vi "Convert_ERDs_Version_ARG.vi"(0 "New Header?":bool, 2 "ERD Name":string[](array[string]), 5 "All_Bundled_Data_Brass":T1, 7 "Array":T8[](array[typedef]) {"ERD Number" format="%.0x"}, 11 "Error In":errorcluster) -> (6 "All_Bundled_Data_Brass 2":T1, 15 "Error Out":errorcluster)   [LabVIEW 2021]
doc: "This VI parses the data from ERDs in correct format, units, etc. It handles all hex to dec conversions, hex to enum, and hex to boolean conversions.\n\nIf Raw Data from ERD is blank string, then it will output values from shift register."
uses:
  Common/LabVIEW GEA2 Toolkit/GEA3/type defs/ERD Read Data Out.ctl
  Type defs/All_Bundled_Data_ARG.ctl
  Common/type defs/Version.ctl
  Common/type defs/CSV_File_String_Arrays.ctl
  Common/type defs/Fault Table Array.ctl
  Common/type defs/Fault_Table_Info.ctl
  Common/type defs/BootloaderVersion.ctl
  Type defs/ERD_Always_Show_ARG.ctl
panel:
  out "Numeric":i32
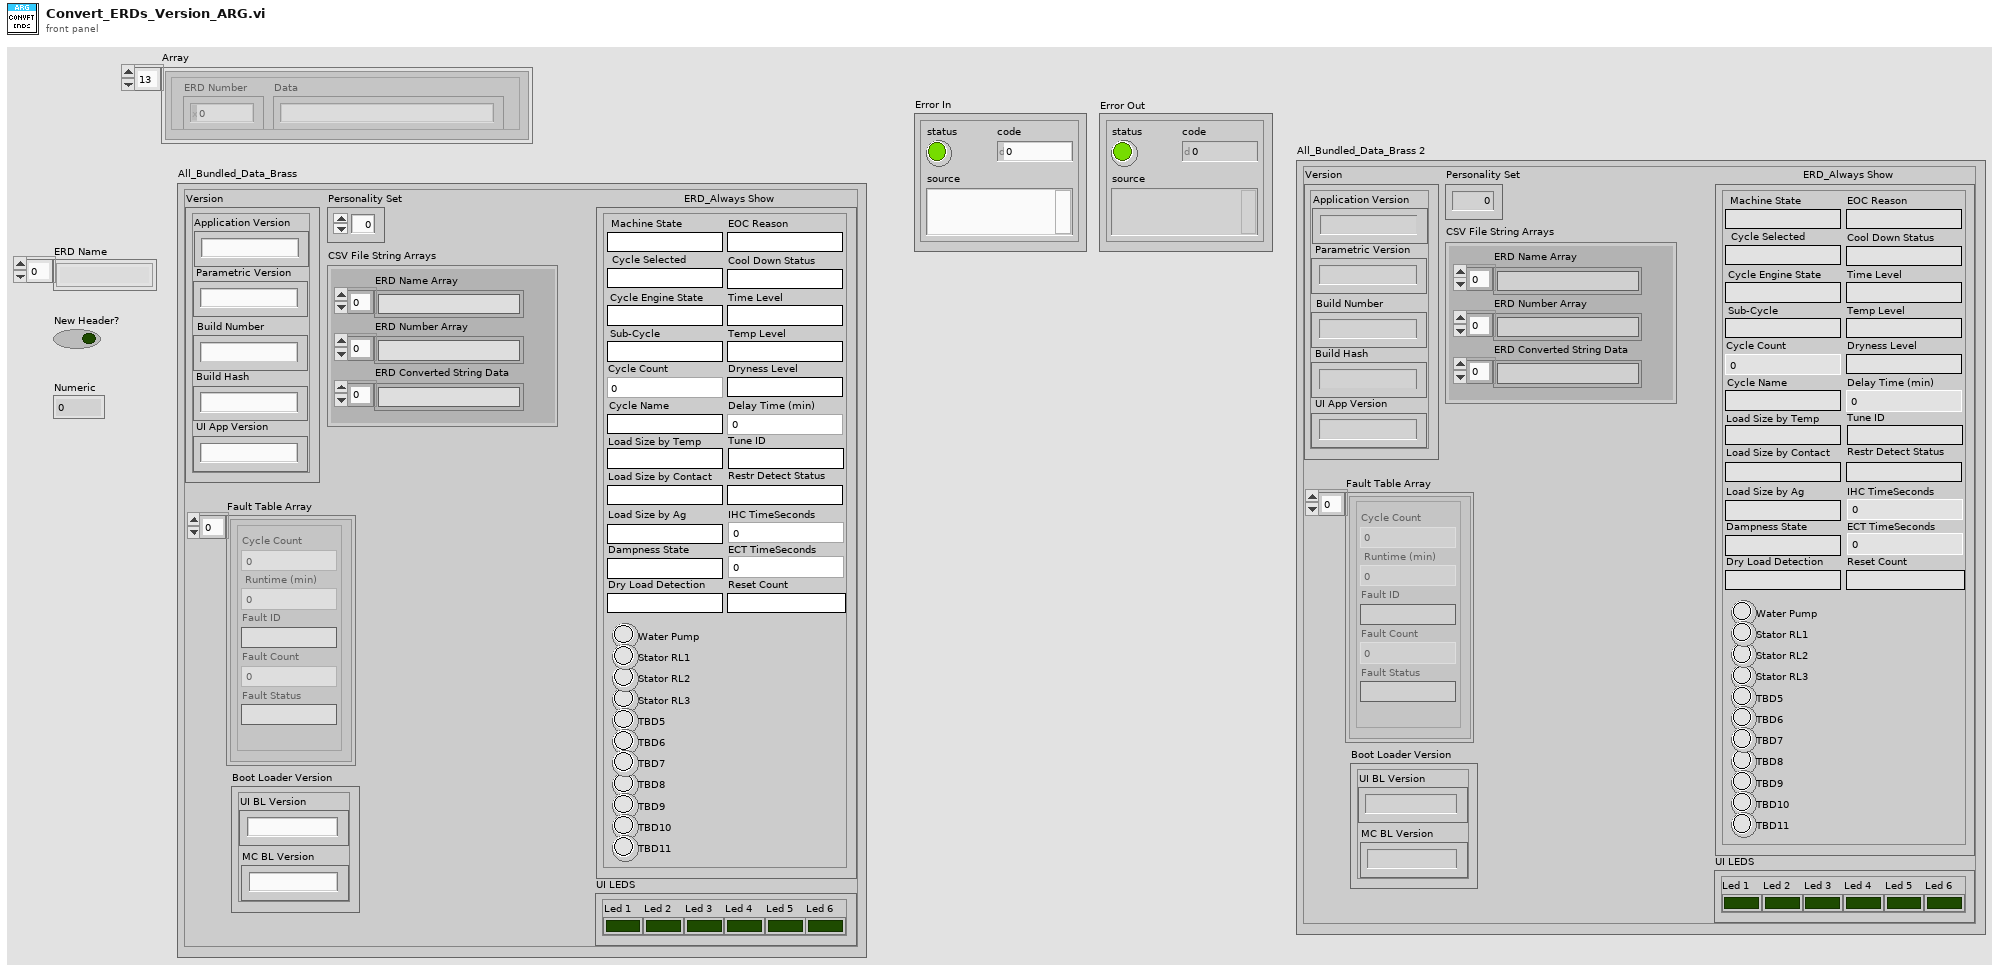
[diagram p1: front panel]
types:
  T1 = typedef "All_Bundled_Data_ARG.ctl" = cluster{"Version":T2, "Personality Set":u8, "CSV File String Arrays":T3, "Fault Table Array ":T4, "Boot Loader Version":T6, "ERD_Always Show":T7, "UI LEDS":cluster{"Led 1":bool, "Led 2":bool, "Led 3":bool, "Led 4":bool, "Led 5":bool, "Led 6":bool}}
  T2 = typedef "Version.ctl" = cluster{"Build Number":string, "Build Hash ":string, "Application Version":string, "Parametric Version":string, "UI App Version":string}
  T3 = typedef "CSV_File_String_Arrays.ctl" = cluster{"ERD Number Array":string[], "ERD Name Array":string[], "ERD Converted String Data":string[]}
  T4 = typedef "Fault Table Array.ctl" = T5[]
  T5 = typedef "Fault_Table_Info.ctl" = cluster{"Cycle Count":u32, " Runtime (min) ":u32, "Fault Status":string, "Fault ID":string, "Fault Count":u16}
  T6 = typedef "BootloaderVersion.ctl" = cluster{"UI BL Version":string, "MC BL Version":string}
  T7 = typedef "ERD_Always_Show_ARG.ctl" = cluster{"Machine State":string, "Cycle Selected":string, "Cycle Engine State":string, "Cycle Count":u32, "Temp Level":string, "Dryness Level":string, "Time Level":string, "Delay Time (min)":u16, "Sub-Cycle":string, "Cycle Name":string, "Tune ID":string, "Restr Detect Status":string, "Load Size by Contact":string, "Load Size by Temp":string, "EOC Reason":string, "Reset Count":string, "Dampness State":string, "Stator RL3":bool, "TBD5":bool, "TBD6":bool, "Water Pump":bool, "Stator RL2":bool, "Cool Down Status":string, "TBD8":bool, "TBD9":bool, "TBD10":bool, "TBD11":bool, "TBD7":bool, "Stator RL1":bool, "IHC TimeSeconds":u32, "ECT TimeSeconds ":u32, "Load Size by Ag":string, "Dry Load Detection":string}
  T8 = typedef "ERD Read Data Out.ctl" = cluster{"ERD Number":u16, "Data":string}
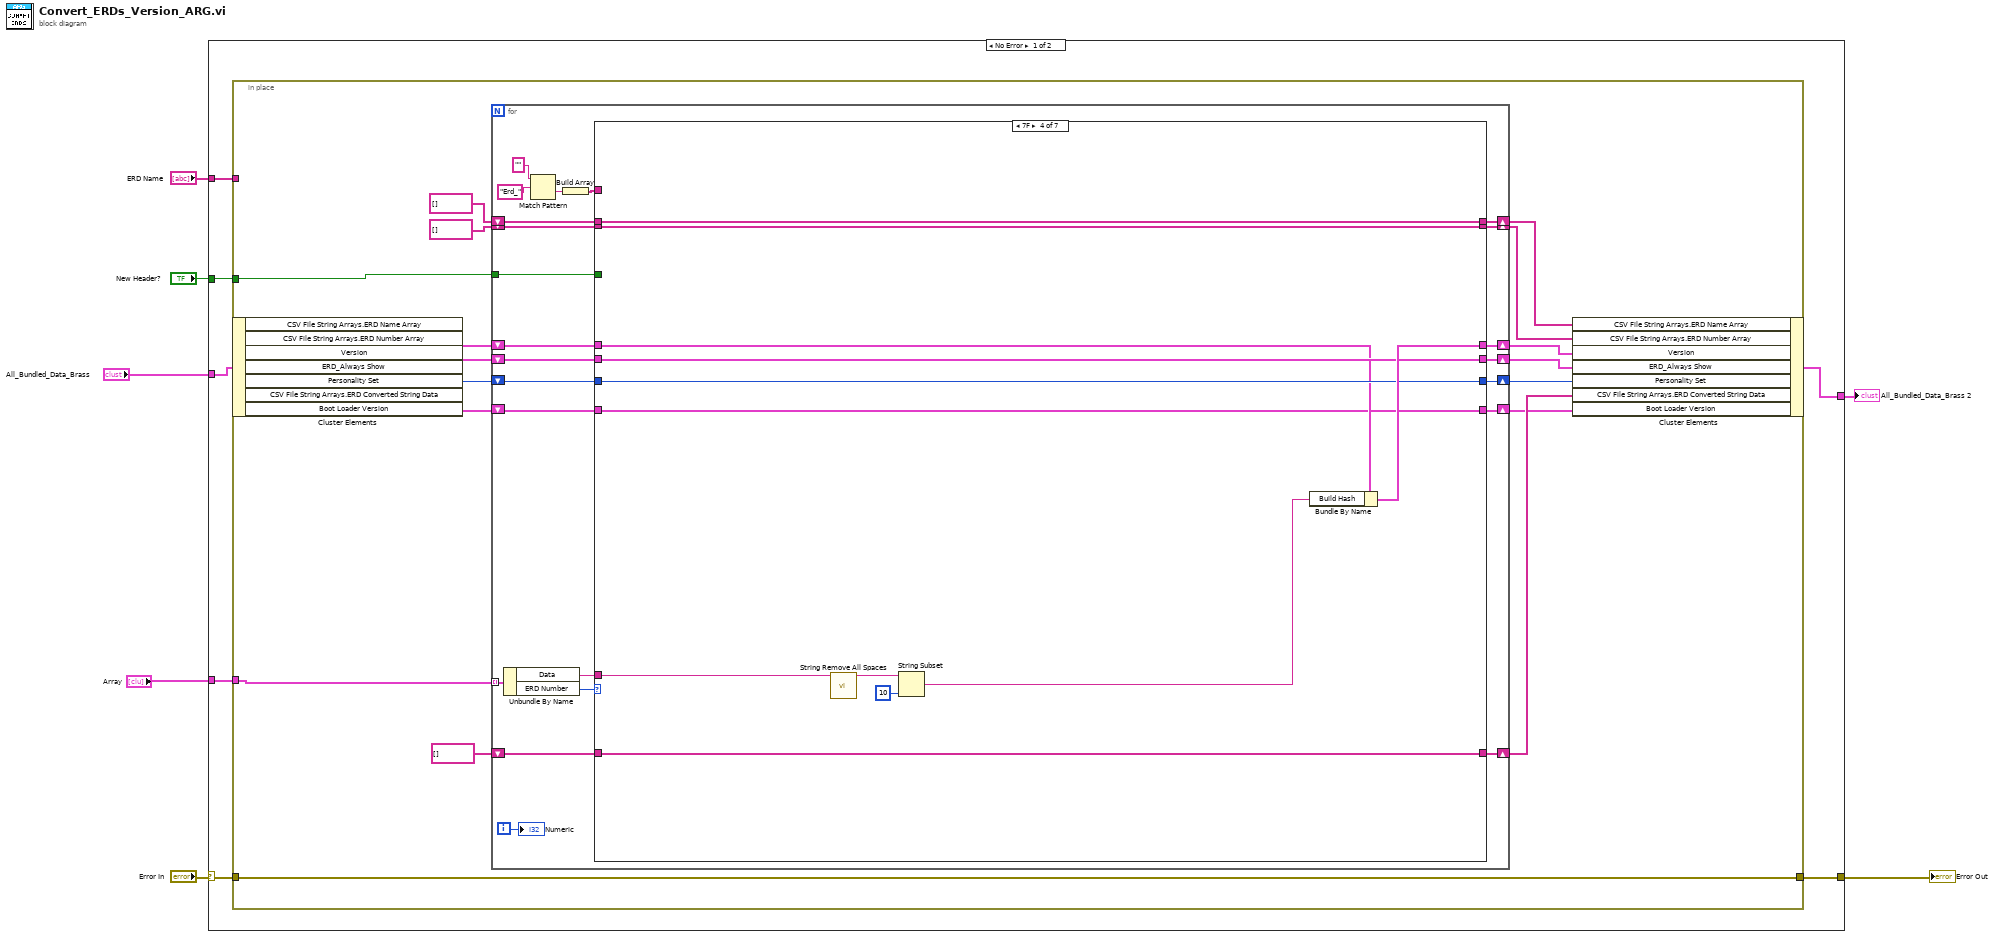
[diagram p0: block diagram]
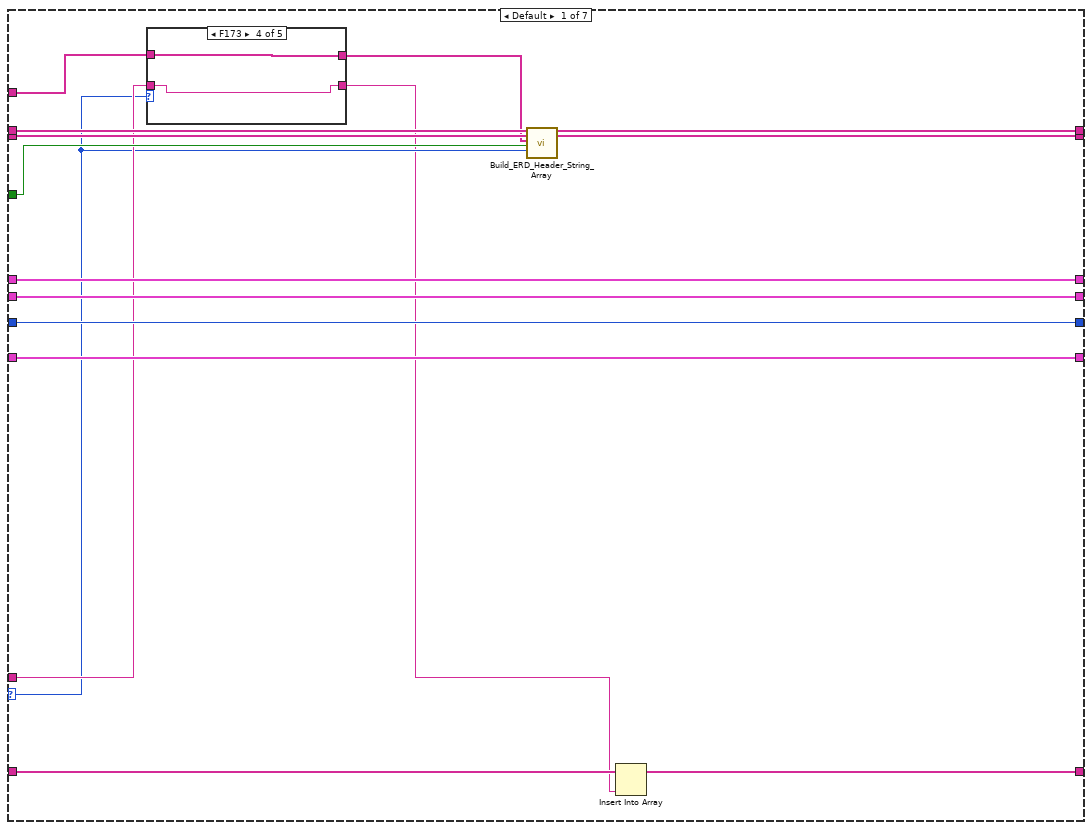
[diagram p2: hidden frame]
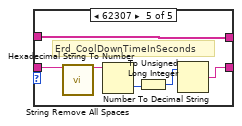
[diagram p6: hidden frame]
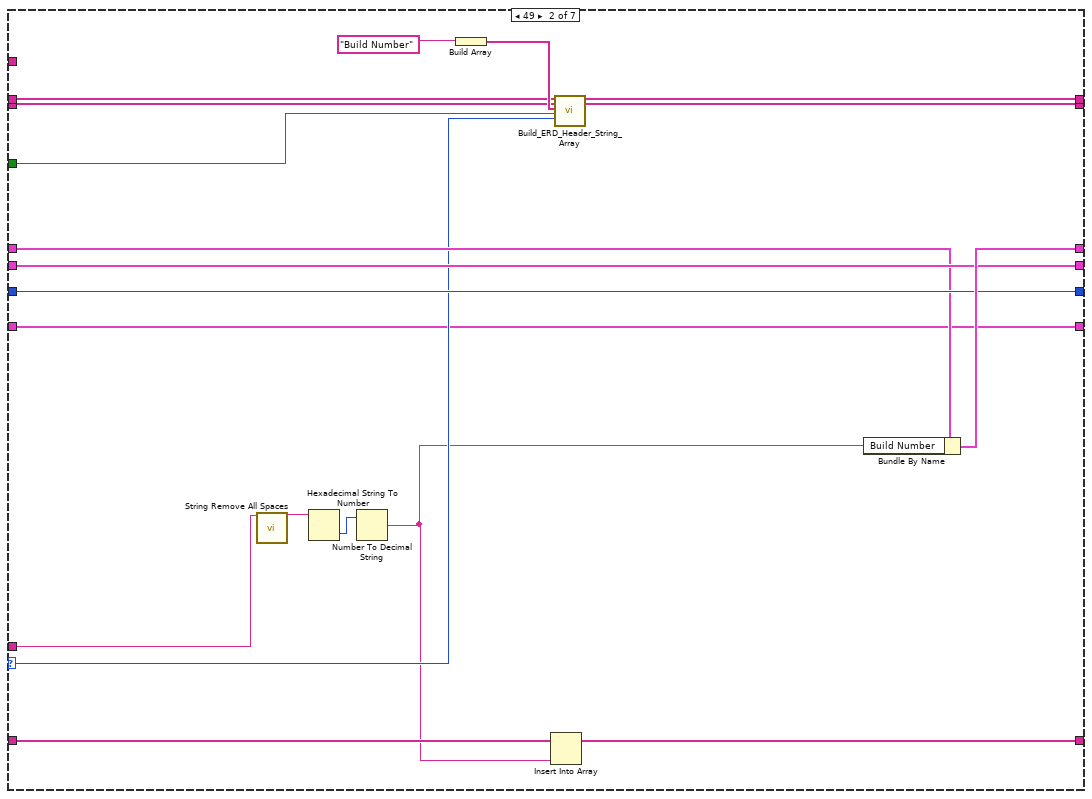
[diagram p7: hidden frame]
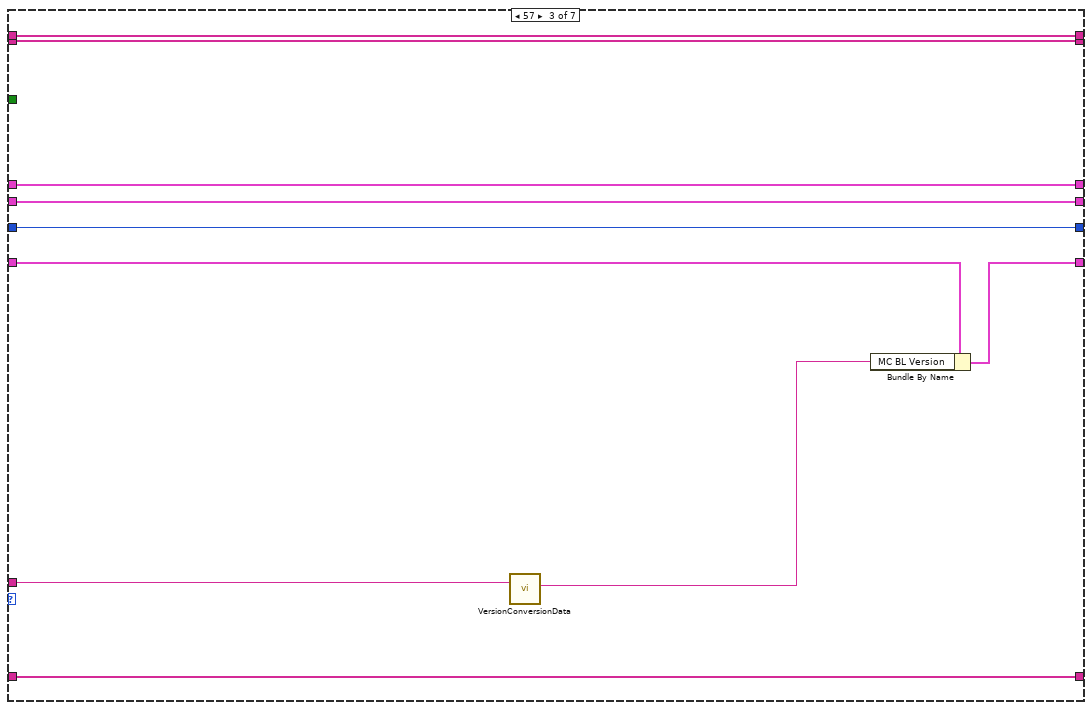
[diagram p8: hidden frame]
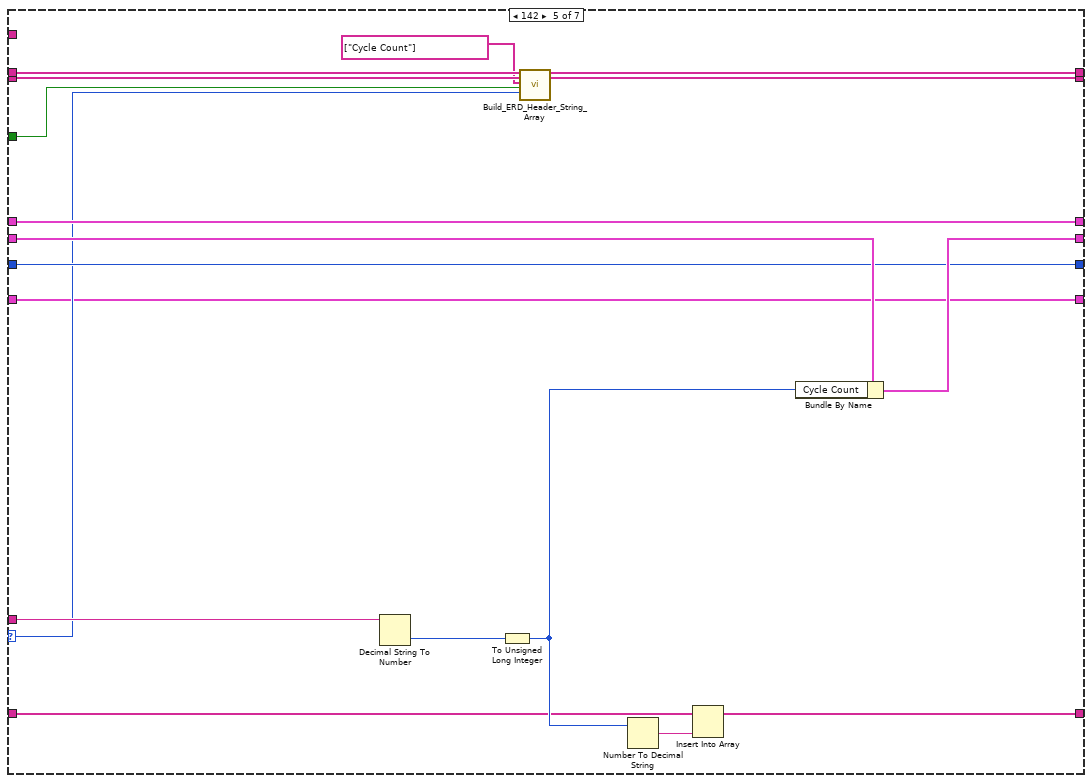
[diagram p9: hidden frame]
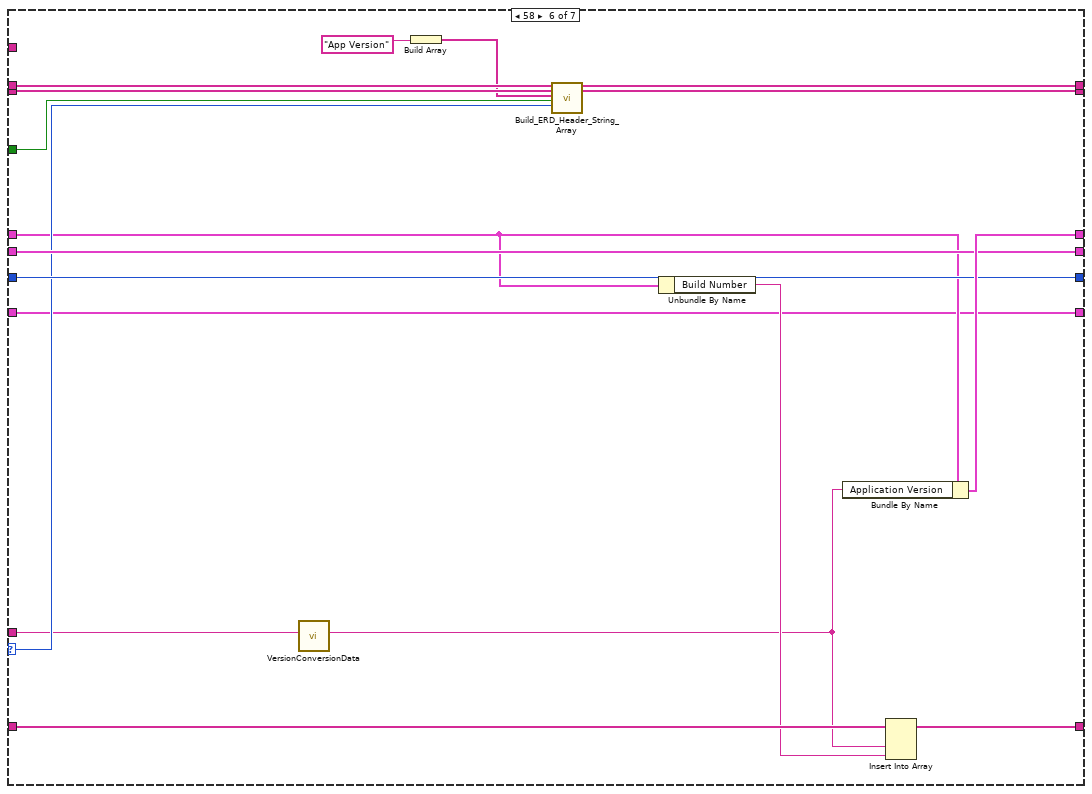
[diagram p10: hidden frame]
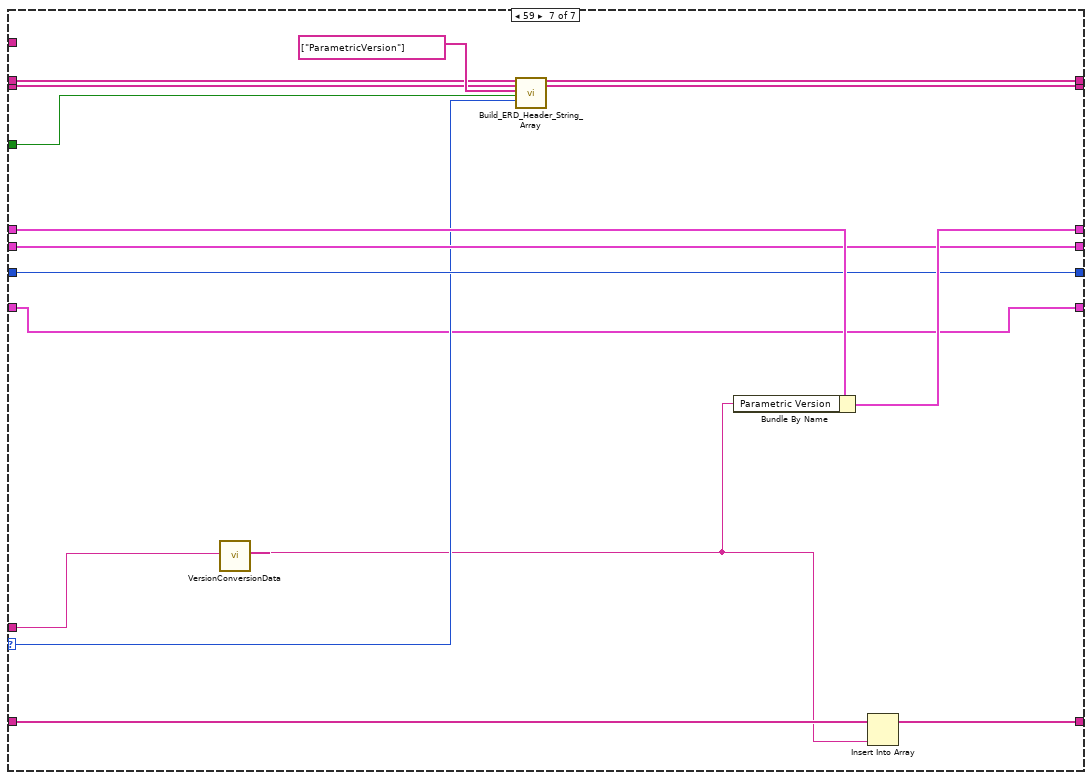
[diagram p11: hidden frame]
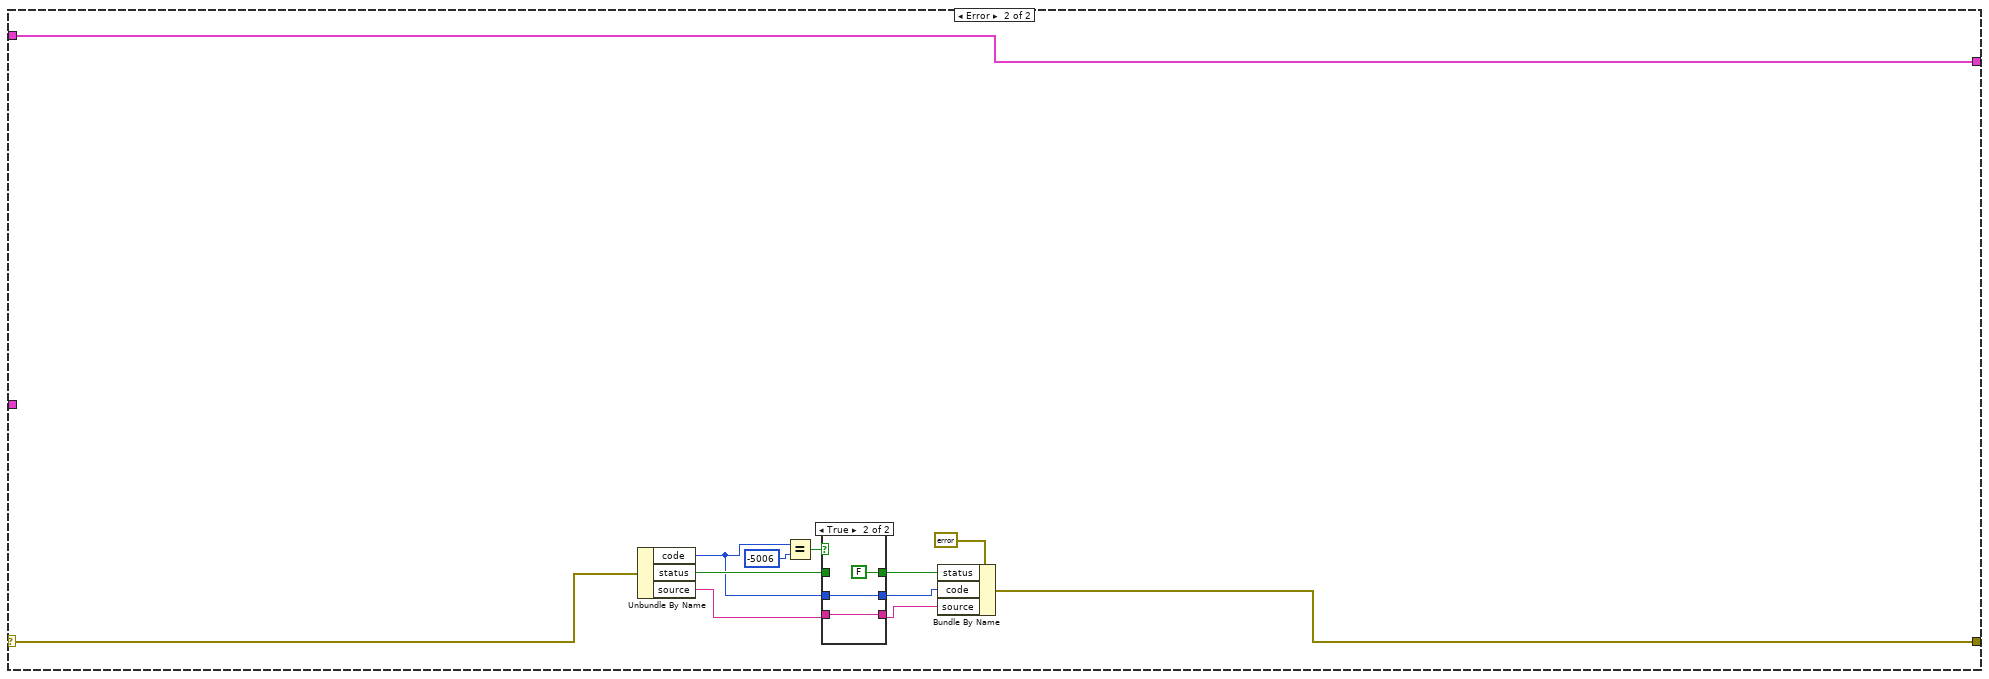
[diagram p12: hidden frame]
diagram:
  n1 = case shown="No Error" "Error In" {
    selector: "Error In" -> [w11 w180]
    tunnel: "Array" -> [w14 _]
    tunnel: [w12 w179] -> w5
    tunnel: "All_Bundled_Data_Brass" -> [w13 w178]
    tunnel: [w10 w178] -> w1
    tunnel: "New Header?" -> [w9 _]
    tunnel: "ERD Name" -> [w8 _]
    frame No Error {
      n2 = in-place {
        in-place-border: w14 -> [w16]
        in-place-border: [w15] -> w12
        in-place-border: w11 -> [w15]
        in-place-border: w9 -> [w24]
        in-place-border: w8 -> [_]
        n3 = in-place-cluster #1(w13) -> ("Version"=w30:T2, "ERD_Always Show"=w31:T7, "Personality Set"=w27:u8, "Boot Loader Version"=w18:T6)  [unwired: 3 out]
        n4 = for {
          shift-right: [w53] -> w28
          shift-left: w31 -> [w52]
          shift-right: [w50] -> w29
          shift-left: w30 -> [w51]
          shift-right: [w47] -> w26
          shift-left: w27 -> [w48]
          shift-right: [w45] -> w19
          shift-left: string[] [] ("ERD String Data") -> [w46]
          tunnel: w24 -> [w44]
          shift-right: [w40] -> w20
          shift-left: string[] [] ("ERD String Data") -> [w43]
          shift-right: [w41] -> w21
          shift-left: string[] [] ("ERD String Data") -> [w42]
          shift-right: [w37] -> w17
          shift-left: w18 -> [w38]
          tunnel: w16 -> [w33] mode=indexing
          i -> [w39]
          n5 = Unbundle By Name(w33) -> ("Data"=w54:string, "ERD Number"=w49:u16)
          n6 = Match Pattern(string="", regular expression="Erd_") -> (after substring=w34:string)  [unwired: 1 in, 3 out]
          n7 = Build Array(w34) -> (w35:string[])
          n8 = case shown="7F" w49 {
            selector: w49 -> [w56 w94 _ _ w132 w153 w165]
            tunnel: w54 -> [w57 w88 w105 w119 w143 w145 w163]
            tunnel: [w70 w102 w113 w124 w141 w160 w175] -> w53
            tunnel: w52 -> [w70 w102 w113 w124 w142 w160 w175]
            tunnel: w51 -> [w69 w100 w106 w120 w140 w152 w177]
            tunnel: [w69 w103 w106 w125 w140 w161 w176] -> w50
            tunnel: w48 -> [w68 w101 w112 w123 w139 w159 w174]
            tunnel: [w68 w101 w112 w123 w139 w159 w174] -> w47
            tunnel: w46 -> [w66 w98 w109 w115 w137 w148 w169]
            tunnel: [w62 w97 w109 w115 w135 w155 w167] -> w45
            tunnel: w44 -> [w64 w92 _ _ w133 w154 w166]
            tunnel: w43 -> [w65 w96 w110 w121 w138 w149 w170]
            tunnel: w42 -> [w60 w90 w111 w122 w128 w158 w173]
            tunnel: [w61 w89 w111 w122 w127 w157 w172] -> w41
            tunnel: [w63 w95 w110 w121 w136 w156 w168] -> w40
            tunnel: w38 -> [w67 w91 w108 w114 w126 w150 w164]
            tunnel: [w67 w91 w107 w114 w126 w150 w164] -> w37
            tunnel: w35 -> [w58 _ _ _ _ _ _]
            frame Default {
              n9 = case shown="F173" w56 {
                tunnel: [w71 w74 w76 w78 w84] -> w59
                tunnel: w58 -> [w71 w74 w76 w78 w84]
                tunnel: w57 -> [w72 w73 w75 w77 w81]
                tunnel: [w72 w73 w75 w77 w79] -> w55
                frame 0, Default {
                  # "ERDs No Data Conversion"
                }
                frame 65423 {
                  # "Consumer Error Mode"
                }
                frame 55 {
                  # "ServiceModeState"
                }
                frame 61811 {
                }
                frame 62307 {
                  # "Erd_CoolDownTimeInSeconds"
                  n10 = call "String Remove All Spaces.vi"("Input String"=w81) -> ("Spaces Removed"=w82:string)  [unwired: 13 in, 1 out]
                  n11 = Hexadecimal String To Number(string=w82) -> (number=w83:u32)  [unwired: 2 in, 1 out]
                  n12 = To Unsigned Long Integer(number=w83) -> (unsigned 32bit integer=w80:u32)
                  n13 = Number To Decimal String(number=w80) -> (decimal integer string=w79:string)  [unwired: 1 in]
                }
              }
              n14 = call "Build_ERD_Header_String_Array.vi"("ERD Name Array In"=w65, "ERD Number Array In"=w66, "ERD Name List"=w59, "New Header?"=w64, "ERD Number"=w56) -> ("ERD Name Array Out"=w63:string[], "ERD Number Array Out"=w62:string[])  [unwired: 13 in]
              n15 = Insert Into Array(array=w60, new element=w55) -> (w61:string[])  [unwired: 1 in]
            }
            frame 49 {
              n16 = call "String Remove All Spaces.vi"("Input String"=w88) -> ("Spaces Removed"=w87:string)  [unwired: 13 in, 1 out]
              n17 = Hexadecimal String To Number(string=w87) -> (number=w85:u32)  [unwired: 2 in, 1 out]
              n18 = Number To Decimal String(number=w85) -> (decimal integer string=w86:string)  [unwired: 1 in]
              n19 = Build Array("Build Number") -> (w99:string[])
              n20 = Insert Into Array(array=w90, new element=w86) -> (w89:string[])  [unwired: 1 in]
              n21 = call "Build_ERD_Header_String_Array.vi"("ERD Name Array In"=w96, "ERD Number Array In"=w98, "ERD Name List"=w99, "New Header?"=w92, "ERD Number"=w94) -> ("ERD Name Array Out"=w95:string[], "ERD Number Array Out"=w97:string[])  [unwired: 13 in]
              n22 = Bundle By Name(cluster=w100, "Build Number"=w86) -> (w103:T2)
            }
            frame 57 {
              n23 = call "VersionConversionData.vi"("Version In"=w105) -> ("Version Out"=w104:string)  [unwired: 9 in, 1 out]
              n24 = Bundle By Name(cluster=w108, "MC BL Version"=w104) -> (w107:T6)
            }
            frame 127 {
              n25 = call "String Remove All Spaces.vi"("Input String"=w119) -> ("Spaces Removed"=w118:string)  [unwired: 13 in, 1 out]
              n26 = String Subset(string=w118, length (rest)=10 ("length (rest)")) -> (substring=w116:string)  [unwired: 1 in]
              n27 = Bundle By Name(cluster=w120, "Build Hash"=w116) -> (w125:T2)
            }
            frame 142 {
              n28 = Decimal String To Number(string=w143) -> (number=w130:i32)  [unwired: 2 in, 1 out]
              n29 = To Unsigned Long Integer(number=w130) -> (unsigned 32bit integer=w129:u32)
              n30 = call "Build_ERD_Header_String_Array.vi"("ERD Name Array In"=w138, "ERD Number Array In"=w137, "ERD Name List"=string[] ["Cycle Count"], "New Header?"=w133, "ERD Number"=w132) -> ("ERD Name Array Out"=w136:string[], "ERD Number Array Out"=w135:string[])  [unwired: 13 in]
              n31 = Number To Decimal String(number=w129) -> (decimal integer string=w131:string)  [unwired: 1 in]
              n32 = Insert Into Array(array=w128, new element=w131) -> (w127:string[])  [unwired: 1 in]
              n33 = Bundle By Name(cluster=w142, "Cycle Count"=w129) -> (w141:T7)
            }
            frame 58 {
              n34 = call "VersionConversionData.vi"("Version In"=w145) -> ("Version Out"=w144:string)  [unwired: 9 in, 1 out]
              n35 = Build Array("App Version" ("String")) -> (w146:string[])
              n36 = call "Build_ERD_Header_String_Array.vi"("ERD Name Array In"=w149, "ERD Number Array In"=w148, "ERD Name List"=w146, "New Header?"=w154, "ERD Number"=w153) -> ("ERD Name Array Out"=w156:string[], "ERD Number Array Out"=w155:string[])  [unwired: 13 in]
              n37 = Unbundle By Name(w152) -> ("Build Number"=w151:string)
              n38 = Bundle By Name(cluster=w152, "Application Version"=w144) -> (w161:T2)
              n39 = Insert Into Array(array=w158, new element #1=w144, new element #2=w151) -> (w157:string[])  [unwired: 1 in]
            }
            frame 59 {
              n40 = call "VersionConversionData.vi"("Version In"=w163) -> ("Version Out"=w162:string)  [unwired: 9 in, 1 out]
              n41 = call "Build_ERD_Header_String_Array.vi"("ERD Name Array In"=w170, "ERD Number Array In"=w169, "ERD Name List"=string[] ["ParametricVersion"], "New Header?"=w166, "ERD Number"=w165) -> ("ERD Name Array Out"=w168:string[], "ERD Number Array Out"=w167:string[])  [unwired: 13 in]
              n42 = Bundle By Name(cluster=w177, "Parametric Version"=w162) -> (w176:T2)
              n43 = Insert Into Array(array=w173, new element=w162) -> (w172:string[])  [unwired: 1 in]
            }
          }
          "Numeric" <- w39
        }
        n44 = in-place-cluster #1("CSV File String Arrays.ERD Name Array"=w20, "CSV File String Arrays.ERD Number Array"=w19, "Version"=w29, "ERD_Always Show"=w28, "Personality Set"=w26, "CSV File String Arrays.ERD Converted String Data"=w21, "Boot Loader Version"=w17) -> (w10:T1)
      }
    }
    frame Error {
      n45 = Unbundle By Name(w180) -> ("code"=w184:i32, "status"=w185:bool, "source"=w182:string)
      n46 = Equal?(x=w184, y=-5006) -> (x = y?=w188:bool)
      n47 = case shown="True" w188 {
        tunnel: [w192 FALSE] -> w186
        tunnel: w185 -> [w192 _]
        tunnel: w184 -> [w191 w194]
        tunnel: [w191 w194] -> w183
        tunnel: [w190 w193] -> w181
        tunnel: w182 -> [w190 w193]
        frame False {
        }
        frame True {
        }
      }
      n48 = Bundle By Name(cluster=errorcluster {"status"=FALSE, "code"=0, "source"=""} ("error constant"), "status"=w186, "code"=w183, "source"=w181) -> (w179:errorcluster)
    }
  }
  "Error Out" <- w5
  "All_Bundled_Data_Brass 2" <- w1
